vi "Write String.vi"(8 "error in (no error)":errorcluster, 10 "String":string, 11 "String Result in":refnum<class "String Result.lvclass">) -> (0 "error out":errorcluster, 3 "String Result out":refnum<class "String Result.lvclass">)   [LabVIEW 2024, in "String Result.lvclass"]
uses:
  String Result.lvclass
  String Result.lvclass/String Result.ctl
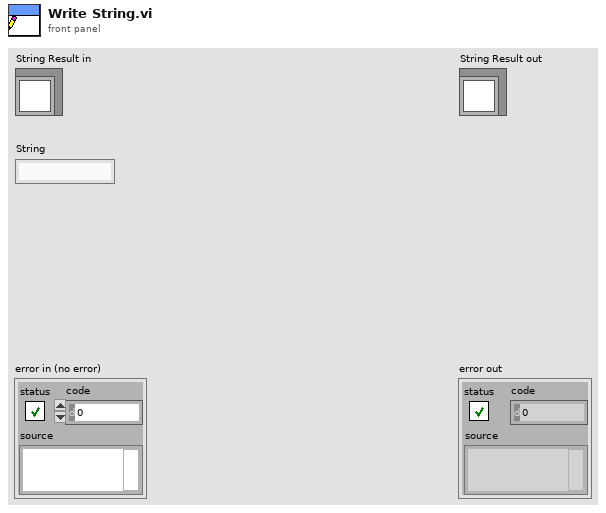
[diagram p1: front panel]
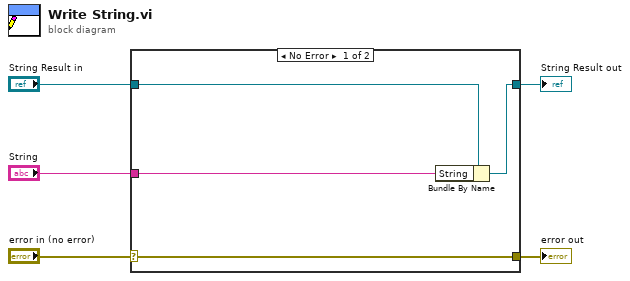
[diagram p0: block diagram]
diagram:
  n1 = case shown="No Error" "error in (no error)" {
    selector: "error in (no error)" -> [w9 w10]
    tunnel: [w9 w10] -> w4
    tunnel: [w7 w11] -> w2
    tunnel: "String Result in" -> [w8 w11]
    tunnel: "String" -> [w6 _]
    frame No Error {
      n2 = Bundle By Name(cluster=w8, "String"=w6) -> (w7:refnum<class "String Result.lvclass">)
    }
    frame Error {
    }
  }
  "error out" <- w4
  "String Result out" <- w2
